vi "Microphone Test.vi"(5 "Test Config":T1={"Chopper RPM"=140, "IR Power"=5, "Conc Tolerance"=0.0, "Gas Stable Time"=0, "A-D Settle"=0, "Samples"=0, "Filter Time"=0, "Gas Mixtures"=[], "Filter Sequences"=[], "Functional Test"={"Mic Test ON ADC Max"=0.0, "Mic Test ON ADC Min"=0.0, "Mic Test OFF ADC Max"=0.0, "Mic Test OFF ADC Min"=0.0, "Mic Test IC ADC Max"=0.0, "Mic Test IC ADC Min"=0.0, "IR Emitter ON ADC Max"=0.0, "IR Emitter ON ADC Min"=0.0, "IR Emitter OFF ADC Max"=0.0, "IR Emitter OFF ADC Min"=0.0}, "Initial Flow Rate"=0.0, "Max Flow Rate"=0.0} {"Gas Mixtures"."ADC Gains" items=["0"=0, "3"=3, "4"=4, "5"=5, "6"=6, "7"=7]; "Conc Tolerance" min=0.0 max=100.0 step=1.0; "IR Power" min=2 max=5 step=1; "Chopper RPM" min=140 max=1000 step=1}, 8 "error in (no error)":errorcluster, 10 "Mic Command":u8, 11 "Session Handle in":T6) -> (0 "error out":errorcluster, 1 "ADC":dbl, 2 "Success?":bool, 3 "Session Handle out":T6)   [LabVIEW 2015, in "PAS.lvclass"]
uses:
  PAS.lvclass
  Typedefs/Session Handle.ctl
  Tests/Controls/Test Config.ctl
  Tests/Controls/Gas Mixture.ctl
  Typedefs/ADC Gains.ctl
  Tests/Controls/Filter Sequence.ctl
  Tests/Controls/Functional Test.ctl
  Typedefs/Emitter Power.ctl
  Typedefs/Valves.ctl
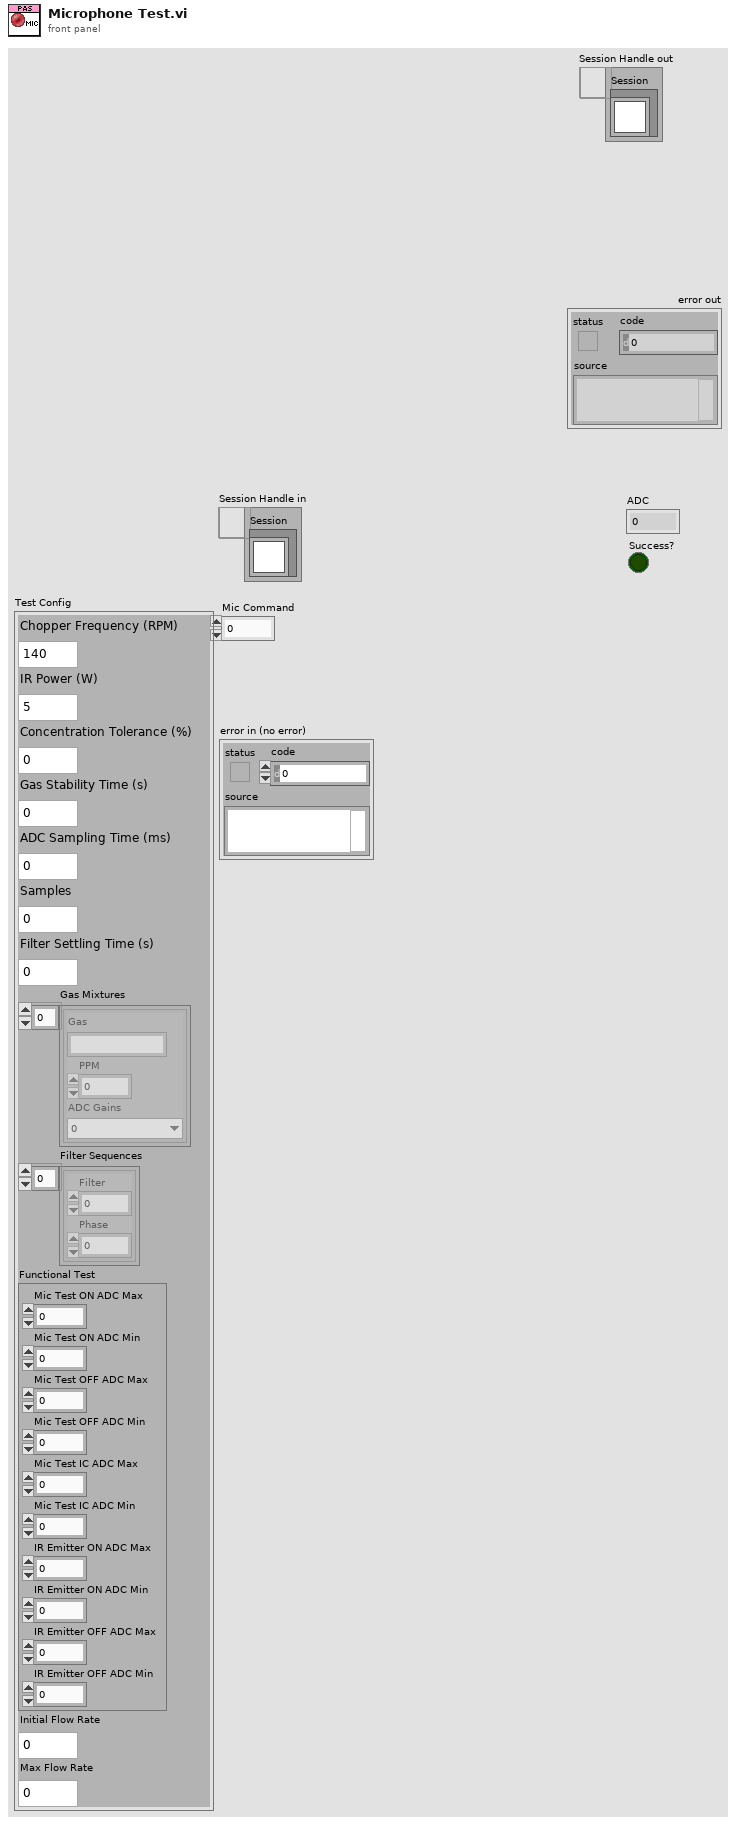
[diagram p1: front panel]
types:
  T1 = typedef "Test Config.ctl" = cluster{"Chopper RPM":u16, "IR Power":u8, "Conc Tolerance":dbl, "Gas Stable Time":u16, "A-D Settle":u16, "Samples":u16, "Filter Time":u16, "Gas Mixtures":T2[], "Filter Sequences":T4[], "Functional Test":T5, "Initial Flow Rate":sgl, "Max Flow Rate":sgl}
  T2 = typedef "Gas Mixture.ctl" = cluster{"Gas":string, "PPM":dbl, "ADC Gains":T3}
  T3 = typedef "PAS.lvclass/ADC Gains.ctl" = u16
  T4 = typedef "Filter Sequence.ctl" = cluster{"Filter":u8, "Phase":dbl}
  T5 = typedef "Functional Test.ctl" = cluster{"Mic Test ON ADC Max":dbl, "Mic Test ON ADC Min":dbl, "Mic Test OFF ADC Max":dbl, "Mic Test OFF ADC Min":dbl, "Mic Test IC ADC Max":dbl, "Mic Test IC ADC Min":dbl, "IR Emitter ON ADC Max":dbl, "IR Emitter ON ADC Min":dbl, "IR Emitter OFF ADC Max":dbl, "IR Emitter OFF ADC Min":dbl}
  T6 = typedef "PAS.lvclass/Session Handle.ctl" = refnum<data-value>
  T7 = typedef "PAS.lvclass/Valves.ctl" = u16
  T8 = typedef "PAS.lvclass/Emitter Power.ctl" = u16
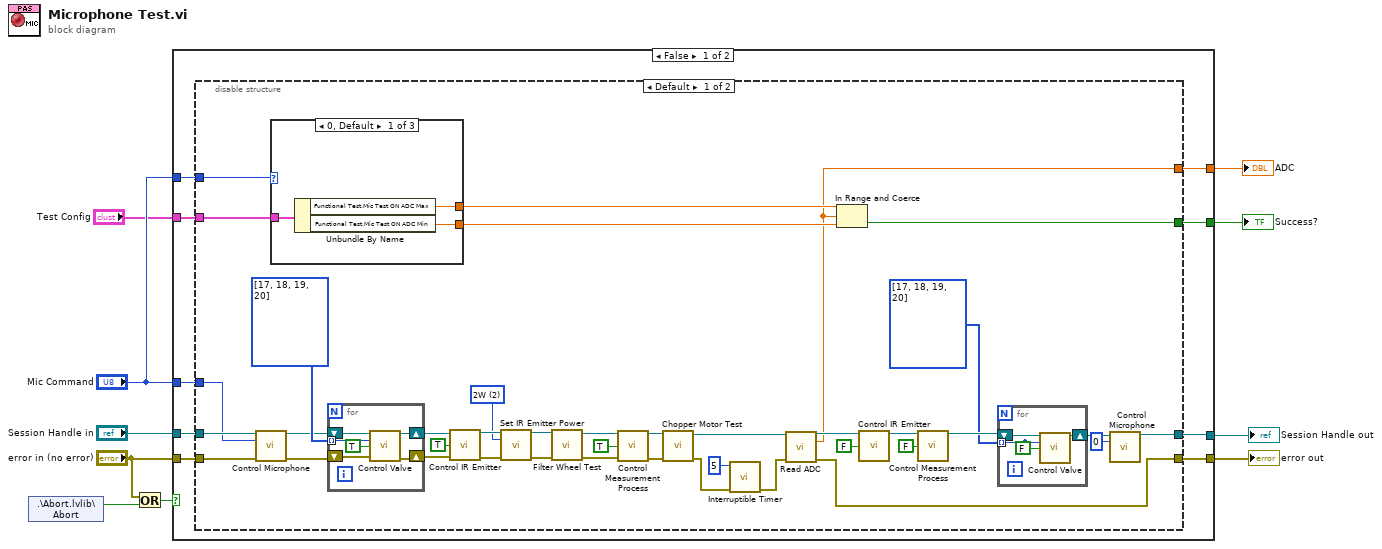
[diagram p0: block diagram]
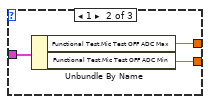
[diagram p2: hidden frame]
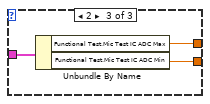
[diagram p3: hidden frame]
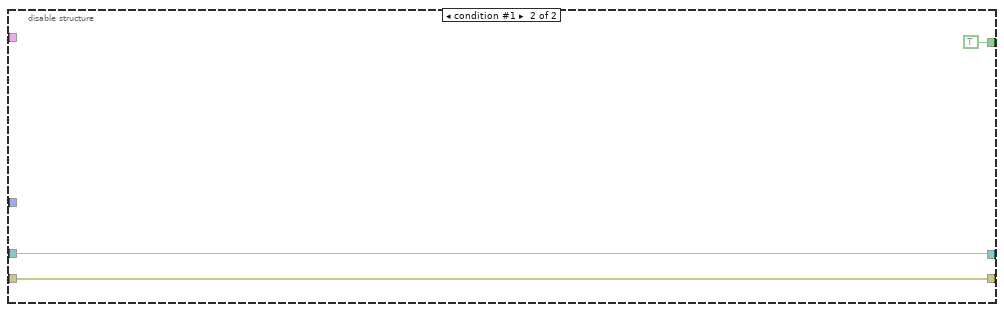
[diagram p4: hidden frame]
diagram:
  n1 = shared-variable ".\\Abort.lvlib\\Abort"() -> (w5:bool)  [unwired: 1 in, 1 out]
  n2 = Or(x="error in (no error)", y=w5) -> (x .or. y?=w7:bool)
  n3 = case shown="False" w7 {
    tunnel: "Test Config" -> [w19 _]
    tunnel: "Session Handle in" -> [w18 w82]
    tunnel: "error in (no error)" -> [w17 w81]
    tunnel: [w11 w82] -> w9
    tunnel: [w16 w81] -> w8
    tunnel: [w15 _] -> w4
    tunnel: [w14 _] -> w3
    tunnel: "Mic Command" -> [w13 _]
    tunnel: "Mic Command" -> [w12 _]
    frame False {
      n4 = disable-structure shown="Default" {
        disable-tunnel: w19 -> [w48 _]
        disable-tunnel: w18 -> [w45 w80]
        disable-tunnel: w17 -> [w44 w79]
        disable-tunnel: [w29 w79] -> w16
        disable-tunnel: [w26 _] -> w15
        disable-tunnel: [w25 TRUE] -> w14
        disable-tunnel: w13 -> [w24 _]
        disable-tunnel: w12 -> [w23 _]
        disable-tunnel: [w21 w80] -> w11
        frame condition #0 (active) {
          w30 = T7[] [17, 18, 19, 20] items=["PV1"=17, "PV2"=18, "PV3"=19, "PV4"=20]
          w52 = T8 2 items=["2W"=2, "3W"=3, "4W"=4, "5W"=5] ("Emitter Power")
          w58 = T7[] [17, 18, 19, 20] items=["PV1"=17, "PV2"=18, "PV3"=19, "PV4"=20]
          n5 = call "Control Microphone.vi"("Session Handle in"=w45, "Command"=w24, "error in (no error)"=w44) -> ("Session Handle out"=w47:T6, "error out"=w46:errorcluster)  [unwired: 9 in, 2 out]
          n6 = case shown="0, Default" w23 {
            tunnel: w48 -> [w61 w64 w67]
            tunnel: [w60 w63 w66] -> w28
            tunnel: [w59 w62 w65] -> w27
            frame 0, Default {
              n7 = Unbundle By Name(w61) -> ("Functional Test.Mic Test ON ADC Max"=w60:dbl, "Functional Test.Mic Test ON ADC Min"=w59:dbl)
            }
            frame 1 {
              n8 = Unbundle By Name(w64) -> ("Functional Test.Mic Test OFF ADC Max"=w63:dbl, "Functional Test.Mic Test OFF ADC Min"=w62:dbl)
            }
            frame 2 {
              n9 = Unbundle By Name(w67) -> ("Functional Test.Mic Test IC ADC Max"=w66:dbl, "Functional Test.Mic Test IC ADC Min"=w65:dbl)
            }
          }
          n10 = for {
            shift-right: [w73] -> w57
            shift-left: w47 -> [w77]
            shift-right: [w74] -> w56
            shift-left: w46 -> [w75]
            tunnel: w58 -> [w76] mode=indexing
            n11 = call "Control Valve.vi"("Session Handle in"=w77, "Valves"=w76, "Energize?"=TRUE, "error in (no error)"=w75) -> ("Session Handle out"=w73:T6, "error out"=w74:errorcluster)  [unwired: 8 in, 2 out]
          }
          n12 = call "Control IR Emitter.vi"("Session Handle in"=w57, "Start?"=TRUE, "error in (no error)"=w56) -> ("Session Handle out"=w54:T6, "error out"=w53:errorcluster)  [unwired: 9 in, 2 out]
          n13 = call "Set IR Emitter Power.vi"("Session Handle in"=w54, "Emitter Power"=w52, "error in (no error)"=w53) -> ("Session Handle out"=w43:T6, "error out"=w42:errorcluster)  [unwired: 10 in, 1 out]
          n14 = call "Filter Wheel Test.vi"("error in (no error)"=w42, "Session Handle in"=w43) -> ("error out"=w40:errorcluster, "Session Handle out"=w41:T6)  [unwired: 7 in, 1 out]
          n15 = call "Control Measurement Process.vi"("Session Handle in"=w41, "Start?"=TRUE, "error in (no error)"=w40) -> ("Session Handle out"=w39:T6, "error out"=w38:errorcluster)  [unwired: 9 in, 2 out]
          n16 = call "Chopper Motor Test.vi"("error in (no error)"=w38, "Session Handle in"=w39) -> ("error out"=w37:errorcluster, "Session Handle out"=w34:T6)  [unwired: 7 in, 1 out]
          n17 = call "Interruptible Timer.vi"("error in (no error)"=w37, "Wait (s)"=5) -> ("error out"=w35:errorcluster)  [unwired: 7 in, 2 out]
          n18 = call "Read ADC.vi"("Session Handle in"=w34, "error in (no error)"=w35) -> ("Session Handle out"=w49:T6, "ADC"=w26:dbl, "error out"=w29:errorcluster)  [unwired: 9 in, 2 out]
          n19 = In Range and Coerce(upper limit=w28, x=w26, lower limit=w27) -> (In Range?=w25:bool)  [unwired: 1 out]
          n20 = call "Control IR Emitter.vi"("Session Handle in"=w49, "Start?"=FALSE) -> ("Session Handle out"=w33:T6)  [unwired: 10 in, 3 out]
          n21 = call "Control Measurement Process.vi"("Session Handle in"=w33, "Start?"=FALSE) -> ("Session Handle out"=w31:T6)  [unwired: 10 in, 3 out]
          n22 = for {
            shift-right: [w70] -> w22
            shift-left: w31 -> [w71]
            tunnel: [w68] -> _ mode=indexing
            tunnel: w30 -> [w68] mode=indexing
            n23 = call "Control Valve.vi"("Session Handle in"=w71, "Valves"=w68, "Energize?"=FALSE) -> ("Session Handle out"=w70:T6)  [unwired: 9 in, 3 out]
          }
          n24 = call "Control Microphone.vi"("Session Handle in"=w22, "Command"=u8 0) -> ("Session Handle out"=w21:T6)  [unwired: 10 in, 3 out]
        }
        frame condition #1 {
        }
      }
    }
    frame True {
    }
  }
  "error out" <- w8
  "Session Handle out" <- w9
  "ADC" <- w4
  "Success?" <- w3
